vi "Open form button constructor.vi"(8 "error in (no error)":errorcluster, 9 "Ctl Refnum":refnum<vi>, 10 "Panel Form":refnum<class "Panel Form Controller.lvclass">, 11 "Open Form Button in":refnum<class "Open Form Button.lvclass">) -> (0 "error out":errorcluster, 3 "Open Form Button out":refnum<class "Open Form Button.lvclass">)   [LabVIEW 2020, in "Panel Form Controller.lvlib" / "Open Form Button.lvclass"]
uses:
  Open Form Button.lvclass
  C:/Users/User/Desktop/Raman Program/Database OOP/source/Database OOP/Button Libraries/Button/Button Class/Button.lvclass
  Form Controller/Panel Form Controller.lvclass
  Database OOP/Button Libraries/Button/Button Class/Button.lvclass/Button.ctl
  Open Form Button.lvclass/Open Form Button.ctl
  Database OOP/Button Libraries/Button/Button Class/Button.lvclass
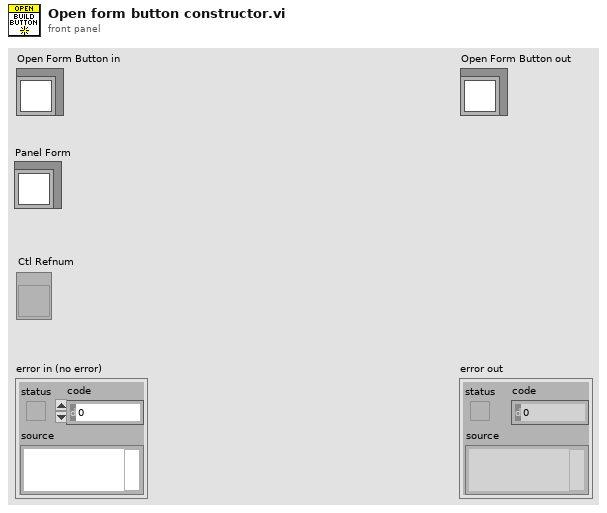
[diagram p1: front panel]
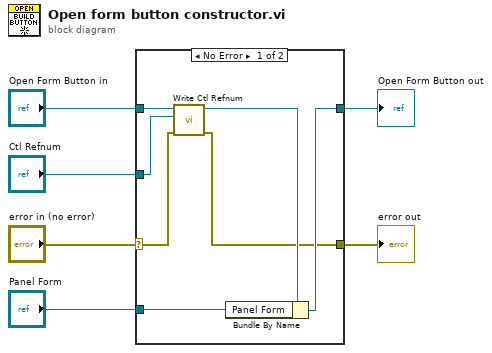
[diagram p0: block diagram]
diagram:
  n1 = case shown="No Error" "error in (no error)" {
    selector: "error in (no error)" -> [w8 w15]
    tunnel: [w7 w15] -> w5
    tunnel: [w11 w14] -> w3
    tunnel: "Open Form Button in" -> [w13 w14]
    tunnel: "Panel Form" -> [w10 _]
    tunnel: "Ctl Refnum" -> [w9 _]
    frame No Error {
      n2 = call "Write Ctl Refnum.vi"("error in (no error)"=w8, "Ctl Refnum"=w9, "Button in"=w13) -> ("error out"=w7:errorcluster, "Button out"=w12:refnum<class "Open Form Button.lvclass">)  [unwired: 7 in]
      n3 = Bundle By Name(cluster=w12, "Panel Form"=w10) -> (w11:refnum<class "Open Form Button.lvclass">)
    }
    frame Error {
    }
  }
  "error out" <- w5
  "Open Form Button out" <- w3
